vi "Type Panel.vi"(11 "TimestampPanel in":refnum<class "TimestampPanel.lvclass">) -> ()   [LabVIEW 2020, in "Conditum-Tools.lvlib" / "TimestampPanel.lvclass"]
uses:
  TimestampPanel.lvclass
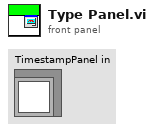
[diagram p1: front panel]
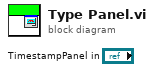
[diagram p0: block diagram]
diagram:
